vi "Data.vi"(7 "LabVIEW Web Service Request":refnum<class "Web Request.lvclass">) -> ()   [LabVIEW 2014]
uses:
  <vilib>/wsapi/Web Request.lvclass
  Reusable/CRDS/Data/Main/CRDS Data.lvclass
  <vilib>/NI/AQ Character Lineator/JSON Serializer/JSON Serializer.lvclass
  <vilib>/NI/AQ Character Lineator/Serializer/Serializer.lvclass
panel:
  out "String":string
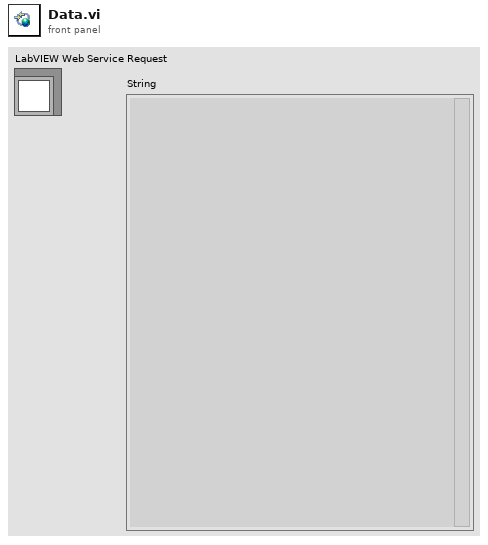
[diagram p1: front panel]
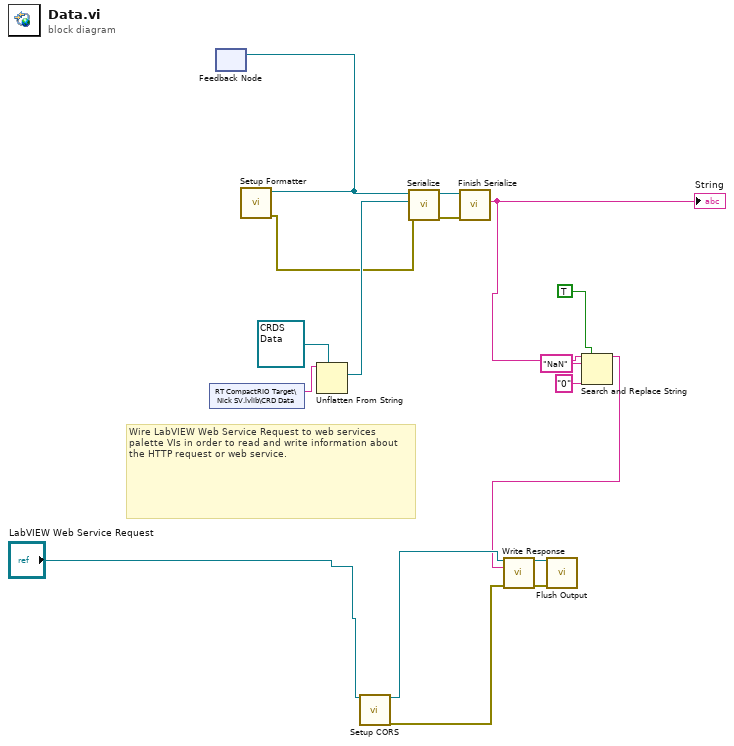
[diagram p0: block diagram]
diagram:
  # "Wire LabVIEW Web Service Request to web services palette VIs in order to read and write information about the HTTP request or web service."
  n1 = shared-variable "RT CompactRIO Target\\Nick SV.lvlib\\CRD Data"() -> (w15:string)  [unwired: 1 in, 1 out]
  n2 = feedback #1() -> ()  [unwired: 2 in]
  n3 = call "Setup Formatter.vi"() -> ("error out"=w9:errorcluster, "JSON Serializer out"=w11:refnum<class "JSON Serializer.lvclass">)  [unwired: 10 in]
  n4 = feedback-in #1(w11) -> ()
  n5 = Unflatten From String(type=refnum<class "CRDS Data.lvclass"> refnum ("CRDS"), binary string=w15) -> (value=w10:refnum<class "CRDS Data.lvclass">)  [unwired: 3 in, 2 out]
  n6 = call "Setup CORS.vi"("Web Request in"="LabVIEW Web Service Request") -> ("Web Request out"=w7:refnum<class "Web Request.lvclass">, "error out"=w6:errorcluster)  [unwired: 17 in]
  n7 = call-dynamic "Serialize.vi"("error in (no error)"=w9, "Serializable"=w10, "JSON Serializer in"=w11) -> ("error out"=w12:errorcluster, "JSON Serializer out"=w13:refnum<class "JSON Serializer.lvclass">)  [unwired: 7 in]
  n8 = call <vilib>:"Finish Serialize.vi"("error in (no error)"=w12, "Serializer in"=w13) -> ("String"=w2:string)  [unwired: 6 in, 3 out]
  "String" <- w2
  n9 = Search and Replace String(replace all?=TRUE ("ignore case? (F)"), input string=w2, search string="NaN", replace string="0" ("replace string (\"\")")) -> (result string=w1:string)  [unwired: 4 in, 3 out]
  n10 = call <vilib>:"Write Response.vi"("LabVIEW Web Service Request"=w7, "response string"=w1, "error in (no error)"=w6) -> ("LabVIEW Web Service Request out"=w17:refnum<class "Web Request.lvclass">, "error out"=w16:errorcluster)  [unwired: 11 in]
  n11 = call <vilib>:"Flush Output.vi"("LabVIEW Web Service Request"=w17, "error in (no error)"=w16) -> ()  [unwired: 12 in, 2 out]
